vi "scanpic2.vi"(8 "error in (no error)":errorcluster, 9 "Size (m)":cluster{"Width":sgl, "Height":sgl}={"Width"=nan, "Height"=nan} caption="Size (m) (NaN=no change)" {"Height" format="%.2p"; "Width" format="%.2p"}, 10 "Application ref in":refnum<vi>, 11 "Center coordinates (m)":cluster{"Xc":sgl, "Yc":sgl}={"Xc"=nan, "Yc"=nan} caption="Center coordinates (m) (NaN=no change)" {"Yc" format="%.2p"; "Xc" format="%.2p"}) -> (0 "Error out":errorcluster, 2 "Application ref out":refnum<vi>, 3 "Data":sgl[][](array[numeric]) format="%#_5p")   [LabVIEW 2020]
uses:
  <userlib>/Nanonis Prog Interface V5/Nanonis Prog Interface.lvlib
panel:
  out "Channel name":string
  in  "Channel index (0-23)":u8
  out "Signals Names":string[](array[string])
  in  "Read channel":i8=14 min=-1
  in  "Pixels":i32 caption="Pixels/line (0=no change)"
  out "Lines":i32
  out "Pixels/line":i32
  out "Channels indexes (0-23)":i32[](array[numeric])
  in  "Serie name":string="ScanMultiBias_"
  in  "Bias increment":sgl=0.1
  out "Bias voltage":sgl caption="Current bias voltage"
  out "Scan":u8 caption="Current scan"
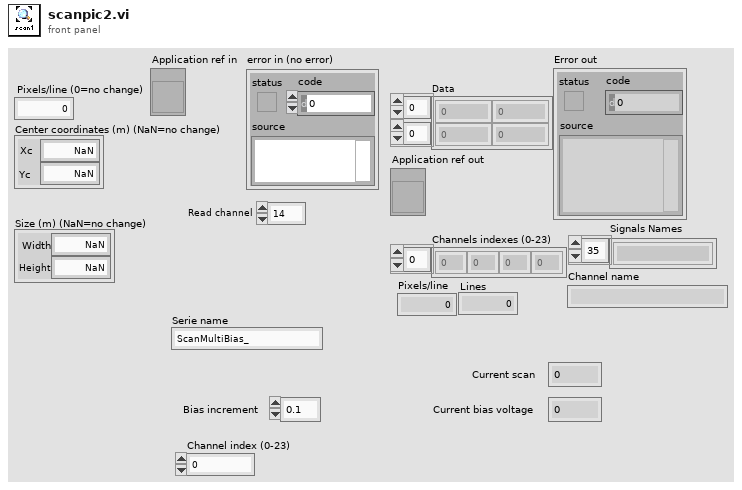
[diagram p1: front panel]
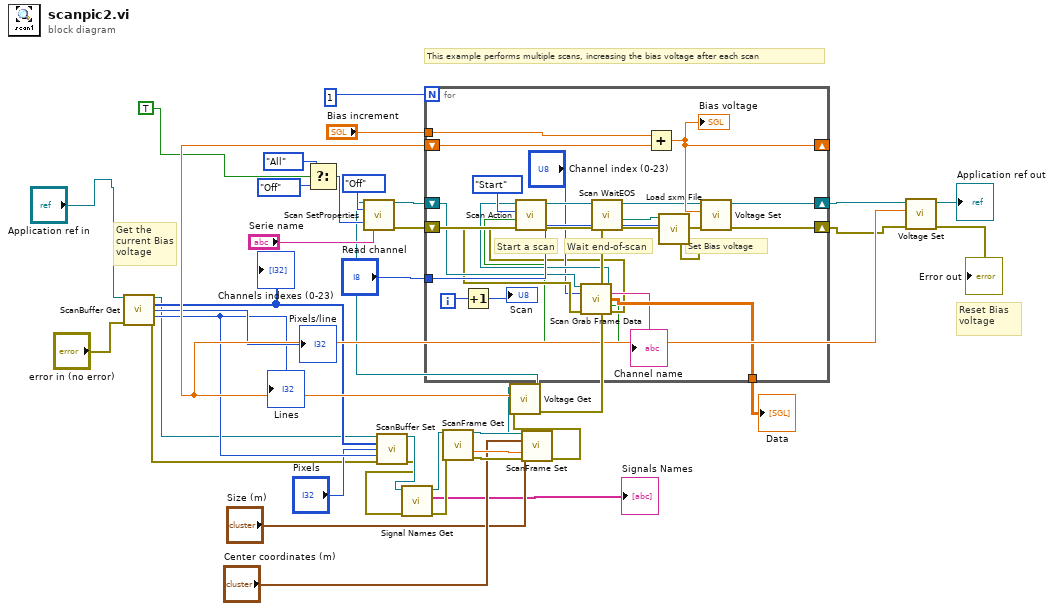
[diagram p0: block diagram]
diagram:
  # "Reset Bias voltage"
  # "This example performs multiple scans, increasing the bias voltage after each scan"
  # "Get the current Bias voltage"
  n1 = call <userlib>:"ScanBuffer Get.vi"("Application ref in"="Application ref in", "error in (no error)"="error in (no error)") -> ("Application ref out"=w2:refnum<vi>, "Channels indexes (0-23)"=w3:i32[], "Pixels/line"=→"Pixels/line":i32, "Lines"=w27:i32, "error out"=w1:errorcluster)  [unwired: 9 in]
  "Channels indexes (0-23)" <- w3
  "Lines" <- w27
  n2 = Select(t=enum16{"No change", "All", "Next", "Off"}."All" ("Auto save"), s=TRUE, f=enum16{"No change", "All", "Next", "Off"}."Off" ("Auto save")) -> (s? t:f=w31:enum16{"No change", "All", "Next", "Off"})
  n3 = call <userlib>:"ScanBuffer Set.vi"("Application ref in"=w2, "Channels indexes (0-23)"=w3, "Pixels"="Pixels", "Lines"=w27, "error in (no error)"=w1) -> ("Application ref out"=w8:refnum<vi>, "error out"=w7:errorcluster)  [unwired: 9 in]
  n4 = call <userlib>:"Signal Names Get.vi"("error in (no error)"=w7, "Application ref in"=w8) -> ("error out"=w5:errorcluster, "Signals Names"=→"Signals Names":string[], "Application ref out"=w6:refnum<vi>)  [unwired: 5 in]
  n5 = call <userlib>:"ScanFrame Get.vi"("Application ref in"=w6, "error in (no error)"=w5) -> ("Application ref out"=w25:refnum<vi>, "Angle (deg)"=w24:sgl, "error out"=w23:errorcluster)  [unwired: 9 in, 2 out]
  n6 = call <userlib>:"ScanFrame Set.vi"("Application ref in"=w25, "Center coordinates (m)"="Center coordinates (m)", "Size (m)"="Size (m)", "Angle (deg)"=w24, "error in (no error)"=w23) -> ("Application ref out"=w21:refnum<vi>, "error out"=w22:errorcluster)  [unwired: 9 in]
  n7 = call <userlib>:"Voltage Get.vi"("error in (no error)"=w22, "Application ref in"=w21) -> ("error out"=w38:errorcluster, "Bias (V)"=w35:sgl, "Application ref out"=w30:refnum<vi>)  [unwired: 7 in]
  n8 = call <userlib>:"Scan SetProperties.vi"("Application ref in"=w30, "Continuous scan"=enum16{"No change", "On", "Off"}."Off", "Auto save"=w31, "Error in (no error)"=w38, "Serie name"="Serie name") -> ("Application ref out"=w29:refnum<vi>, "Error out"=w37:errorcluster)  [unwired: 9 in]
  n9 = for {
    N: 1 -> [_]
    tunnel: "Bias increment" -> [w62]
    shift-right: [w61] -> w18
    shift-left: w37 -> [w44]
    shift-right: [w56] -> _
    shift-left: w35 -> [w57]
    shift-right: [w52] -> w17
    shift-left: w29 -> [w46]
    tunnel: "Read channel" -> [w50]
    tunnel: [w47] -> w15
    i -> [w60]
    # "Set Bias voltage"
    # "Wait end-of-scan"
    # "Start a scan"
    n10 = Increment(x=w60) -> (x+1=→"Scan":i32)
    n11 = call <userlib>:"Scan Grab Frame Data.vi"("Application ref in"=w46, "Channel index (0-23)"="Channel index (0-23)", "error in (no error)"=w44) -> ("Application ref out"=w45:refnum<vi>, "Channel name"=→"Channel name":string, "Scan frame data"=w47:sgl[][], "Direction: up/down (T=up)"=w40:bool, "error out"=w41:errorcluster)  [unwired: 8 in]
    n12 = call <userlib>:"Scan Action.vi"("error in (no error)"=w41, "Direction: up/down (T=up)"=w40, "Scan action (Start)"=enum16{"Start", "Stop", "Pause", "Resume"}."Start" ("Scan action"), "Application ref in"=w45) -> ("error out"=w58:errorcluster, "Application ref out"=w54:refnum<vi>)  [unwired: 5 in]
    n13 = call <userlib>:"Scan WaitEOS.vi"("error in (no error)"=w58, "Application ref in"=w54) -> ("error out"=w49:errorcluster, "Saved file path"=w51:path, "Application ref out"=w53:refnum<vi>)  [unwired: 5 in, 1 out]
    n14 = Add(x=w62, y=w57) -> (x+y=w56:sgl)
    "Bias voltage" <- w56
    n15 = call <userlib>:"Load sxm File.vi"("error in"=w49, "Read channel"=w50, "Scan data file"=w51) -> ("error out"=w48:errorcluster)  [unwired: 3 in, 5 out]
    n16 = call <userlib>:"Voltage Set.vi"("Error in (no error)"=w48, "Bias (V)"=w56, "Application ref in"=w53) -> ("Error out"=w61:errorcluster, "Application ref out"=w52:refnum<vi>)  [unwired: 7 in]
  }
  "Data" <- w15
  n17 = call <userlib>:"Voltage Set.vi"("Error in (no error)"=w18, "Bias (V)"=w35, "Application ref in"=w17) -> ("Error out"=→"Error out":errorcluster, "Application ref out"=→"Application ref out":refnum<vi>)  [unwired: 7 in]
